vi "LJStreamM build log data string.vi"(4 "Scan Rate":dbl=50.0 format="%.2f", 6 "Time":dbl format="%.2f", 8 "Disable Scaling":bool, 9 "Scaled Data":dbl[][](array[numeric]) format="%.3f", 10 "Raw Data":dbl[][](array[numeric]) format="%.3f") -> (3 "Output data":string)   [LabVIEW 2026]
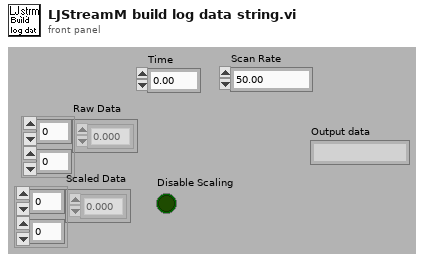
[diagram p1: front panel]
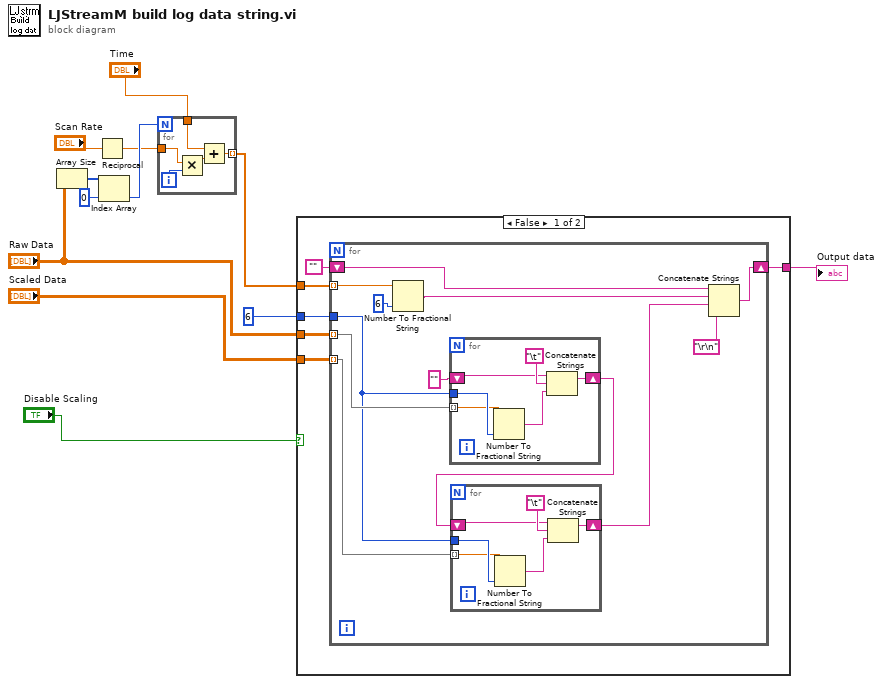
[diagram p0: block diagram]
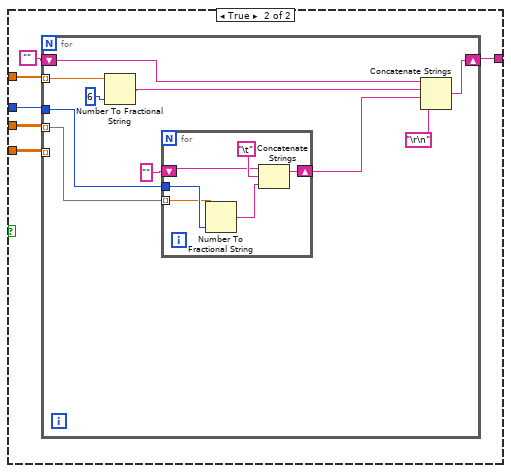
[diagram p2: hidden frame]
diagram:
  n1 = Array Size(array="Raw Data") -> (size(s)=w12:i32[])
  n2 = Reciprocal(x="Scan Rate") -> (1/x=w7:dbl)
  n3 = Index Array(array=w12, index=0 ("Index")) -> (element=w10:i32)
  n4 = for {
    N: w10 -> [_]
    tunnel: "Time" -> [w17]
    tunnel: w7 -> [w13]
    tunnel: [w16] -> w6 mode=indexing
    i -> [w14]
    n5 = Multiply(x=w13, y=w14) -> (x*y=w15:dbl)
    n6 = Add(x=w17, y=w15) -> (x+y=w16:dbl)
  }
  n7 = case shown="False" "Disable Scaling" {
    tunnel: w6 -> [w23 w49]
    tunnel: "Raw Data" -> [w22 w51]
    tunnel: "Scaled Data" -> [w21 w52]
    tunnel: [w20 w48] -> w1
    tunnel: i16 6 ("precision (6)") -> [w19 w50]
    frame False {
      n8 = for {
        shift-right: [w31] -> w20
        shift-left: "" -> [w32]
        tunnel: w23 -> [w34] mode=indexing
        tunnel: w22 -> [w29] mode=indexing
        tunnel: w21 -> [w24] mode=indexing
        tunnel: w19 -> [w25]
        n9 = Number To Fractional String(number=w34, precision (6)=i16 6) -> (F-format string=w33:string)  [unwired: 2 in]
        n10 = for {
          shift-right: [w45] -> w27
          shift-left: "" -> [w46]
          tunnel: w25 -> [w43]
          tunnel: w29 -> [w42] mode=indexing
          n11 = Number To Fractional String(number=w42, precision (6)=w43) -> (F-format string=w44:string)  [unwired: 2 in]
          n12 = Concatenate Strings(w46, "\t", w44) -> (w45:string)
        }
        n13 = for {
          shift-right: [w39] -> w26
          shift-left: w27 -> [w40]
          tunnel: w25 -> [w37]
          tunnel: w24 -> [w36] mode=indexing
          n14 = Number To Fractional String(number=w36, precision (6)=w37) -> (F-format string=w38:string)  [unwired: 2 in]
          n15 = Concatenate Strings(w40, "\t", w38) -> (w39:string)
        }
        n16 = Concatenate Strings(w32, w33, w26, "\r\n") -> (w31:string)
      }
    }
    frame True {
      n17 = for {
        shift-right: [w59] -> w48
        shift-left: "" -> [w60]
        tunnel: w49 -> [w62] mode=indexing
        tunnel: w51 -> [w57] mode=indexing
        tunnel: w52 -> [_] mode=indexing
        tunnel: w50 -> [w55]
        n18 = Number To Fractional String(number=w62, precision (6)=i16 6) -> (F-format string=w61:string)  [unwired: 2 in]
        n19 = for {
          shift-right: [w67] -> w54
          shift-left: "" -> [w68]
          tunnel: w55 -> [w65]
          tunnel: w57 -> [w64] mode=indexing
          n20 = Number To Fractional String(number=w64, precision (6)=w65) -> (F-format string=w66:string)  [unwired: 2 in]
          n21 = Concatenate Strings(w68, "\t", w66) -> (w67:string)
        }
        n22 = Concatenate Strings(w60, w61, w54, "\r\n") -> (w59:string)
      }
    }
  }
  "Output data" <- w1
